vi "Find APU.vi"(8 "error in (no error)":errorcluster, 10 "Name":string, 11 "EST Custom Device in":refnum<k24>) -> (0 "error out":errorcluster, 2 "APU":refnum<k24>, 3 "EST Custom Device out":refnum<k24>)   [LabVIEW 2019, in "Engine Simulation Toolkit Scripting API.lvlib"]
uses:
  Engine Simulation Toolkit Scripting API.lvlib
  NationalInstruments.VeriStand.SystemDefinitionAPI
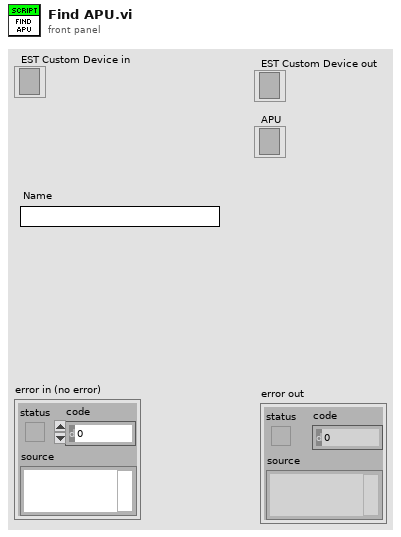
[diagram p1: front panel]
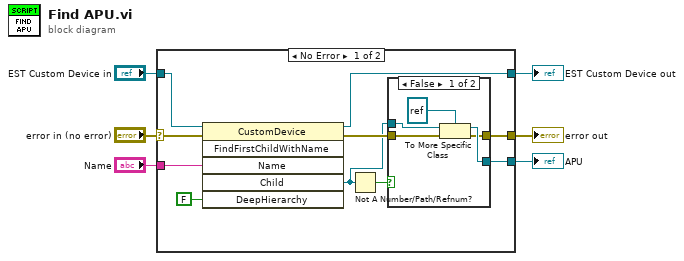
[diagram p0: block diagram]
diagram:
  n1 = case shown="No Error" "error in (no error)" {
    selector: "error in (no error)" -> [w13 w24]
    tunnel: [w9 w24] -> w6
    tunnel: "EST Custom Device in" -> [w16 w23]
    tunnel: [w14 w23] -> w3
    tunnel: "Name" -> [w15 _]
    tunnel: [w11 _] -> w1
    frame No Error {
      n2 = invoke class="CustomDevice" method="FindFirstChildWithName"(reference=w16, error in=w13, "Name"=w15, "DeepHierarchy"=FALSE) -> (reference out=w14:refnum<k24>, error out=w10:errorcluster, "Child"=w8:refnum<k24>)  [unwired: 2 in, 3 out]
      n3 = Not A Number/Path/Refnum?(number/path/refnum=w8) -> (NaN/Path/Refnum?=w7:bool)
      n4 = case shown="False" w7 {
        tunnel: [w21 _] -> w11
        tunnel: w10 -> [w20 w22]
        tunnel: [w19 w22] -> w9
        tunnel: w8 -> [w17 _]
        frame False {
          n5 = To More Specific Class(target class=refnum<k24> refnum ("APU"), reference=w17, error in=w20) -> (specific class reference=w21:refnum<k24>, error out=w19:errorcluster)
        }
        frame True {
        }
      }
    }
    frame Error {
    }
  }
  "EST Custom Device out" <- w3
  "error out" <- w6
  "APU" <- w1
